vi "_Obtain SyncStart Queue.vi"(11 "Name(\"\" to use topmostVI Name)":string) -> (0 "error out":errorcluster, 3 "Queue out":refnum<queue>)   [LabVIEW 2017, in "SyncStart.lvlib"]
uses:
  SyncStart.lvlib
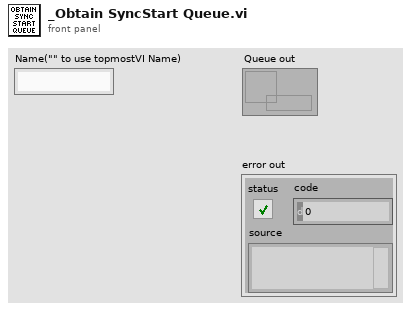
[diagram p1: front panel]
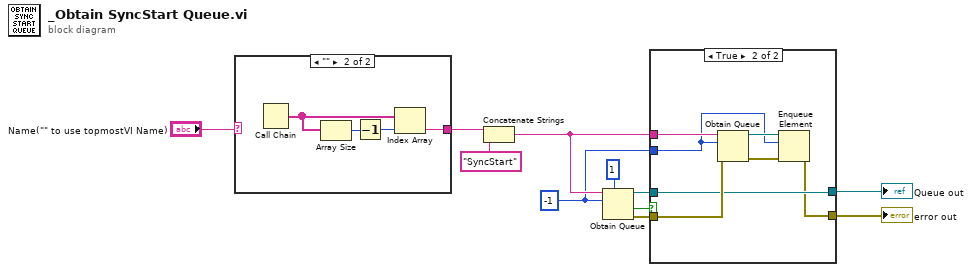
[diagram p0: block diagram]
diagram:
  w8 = -1 ("create if not found? (T)")
  n1 = case shown="\"\"" "Name(\"\" to use topmostVI Name)" {
    selector: "Name(\"\" to use topmostVI Name)" -> [w12 _]
    tunnel: [w12 w13] -> w4
    frame "False", Default {
    }
    frame "" {
      n2 = Call Chain() -> (call chain=w15:string[])
      n3 = Array Size(array=w15) -> (size(s)=w16:i32)
      n4 = Decrement(x=w16) -> (x-1=w14:i32)
      n5 = Index Array(array=w15, index=w14) -> (element=w13:string)
    }
  }
  n6 = Concatenate Strings(w4, "SyncStart" ("string")) -> (w9:string)
  n7 = Obtain Queue(max queue size (-1, unlimited)=1, name (unnamed)=w9, element data type=w8) -> (queue out=w3:refnum<queue>, created new?=w2:bool, error out=w5:errorcluster)  [unwired: 2 in]
  n8 = case shown="True" w2 {
    tunnel: w3 -> [w18 w21]
    tunnel: [w18 w21] -> w6
    tunnel: w9 -> [_ w23]
    tunnel: w5 -> [w17 w22]
    tunnel: [w17 w20] -> w7
    tunnel: w8 -> [_ w19]
    frame False {
    }
    frame True {
      n9 = Obtain Queue(name (unnamed)=w23, element data type=w19, error in (no error)=w22) -> (queue out=w25:refnum<queue>, error out=w24:errorcluster)  [unwired: 2 in, 1 out]
      n10 = Enqueue Element(queue=w25, element=w19, error in (no error)=w24) -> (error out=w20:errorcluster)  [unwired: 1 in, 2 out]
    }
  }
  "error out" <- w7
  "Queue out" <- w6
